vi "FlowPID.vi"() -> ()   [LabVIEW 2017]
uses:
  BERTTA.dll
panel:
  out "output2":dbl
  out "amount_out":dbl
  in  "flow_in":dbl
  out "errsum":i32
  out "Waveform Chart":dynamicdata(graph)
  out "error":i32
  out "output":i32
  out "timechange":i32
  out "lastTime":i32
  in  "kd":dbl
  in  "ki":dbl=1e-05
  in  "kp":dbl=0.001
  in  "Setpoint":dbl=2000.0
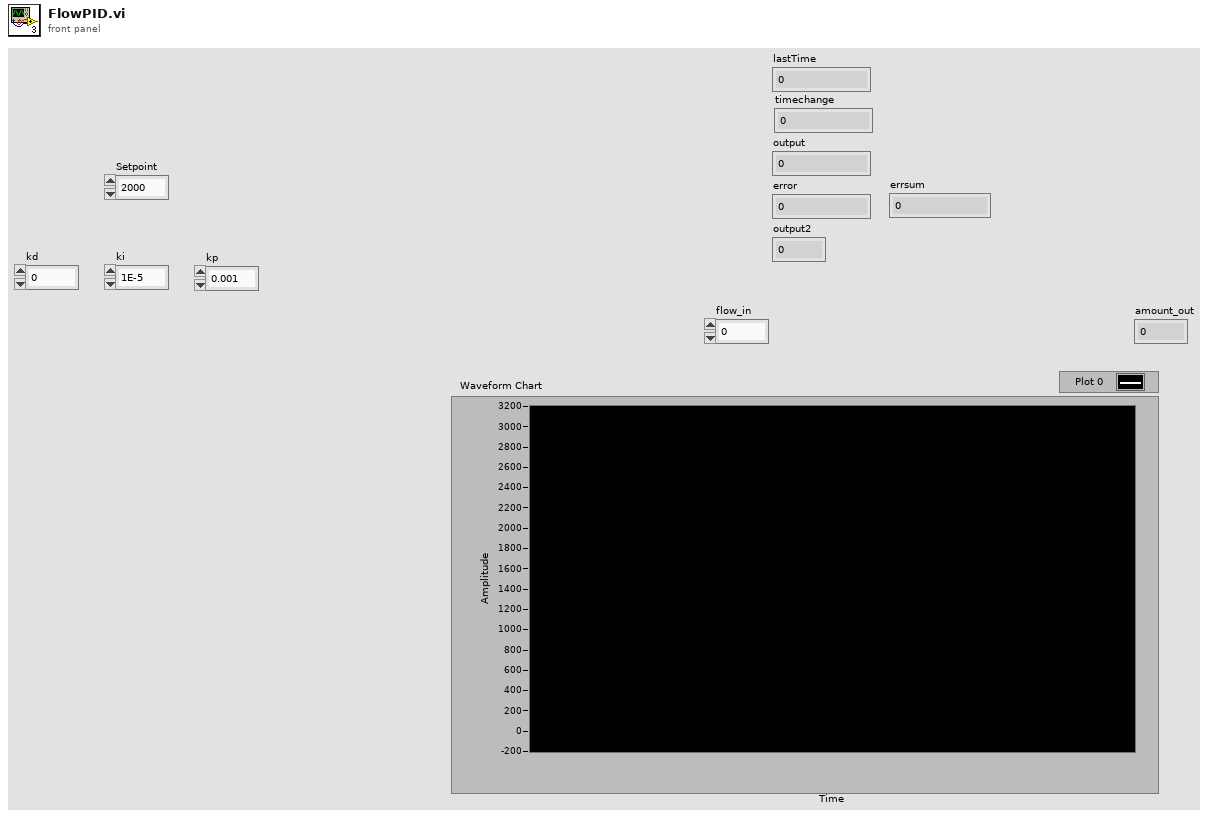
[diagram p1: front panel]
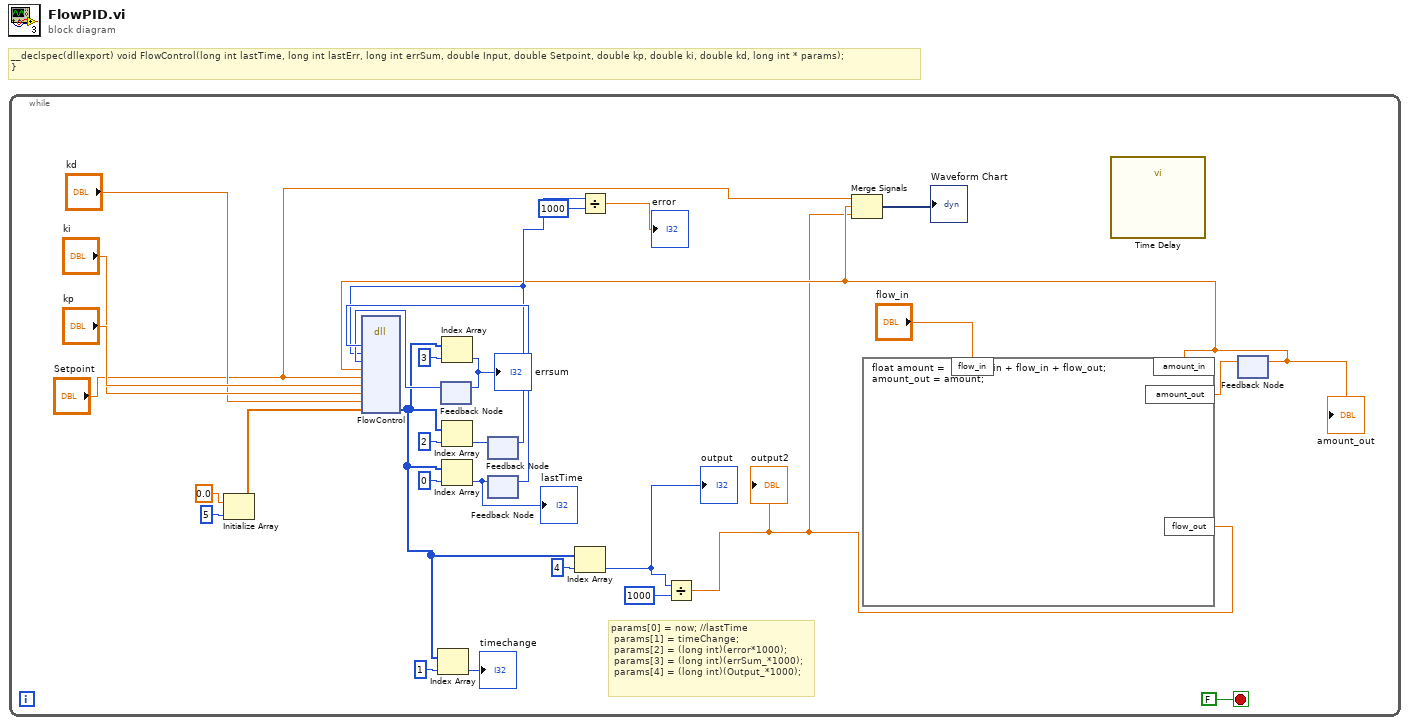
[diagram p0: block diagram]
diagram:
  # "__declspec(dllexport) void FlowControl(long int lastTime, long int lastErr, long int errSum, double Input, double Setpoint, double kp, double ki, double kd, long int * params);\n}"
  n1 = while {
    stop <- FALSE stop-if-true
    # "params[0] = now; //lastTime\n\tparams[1] = timeChange;\n\tparams[2] = (long int)(error*1000);\n\tparams[3] = (long int)(errSum_*1000);\n\tparams[4] = (long int)(Output_*1000);"
    n2 = Initialize Array(0.0 ("element"), 5 ("dimension size")) -> (w27:dbl[])
    n3 = feedback #1() -> (w14:i32)  [unwired: 1 in]
    n4 = feedback #2() -> (w11:i32)  [unwired: 1 in]
    n5 = feedback #3() -> (w20:i32)  [unwired: 1 in]
    n6 = Divide(x=w11, y=1000) -> (x/y=→"error":dbl)
    n7 = call "Time Delay"() -> ()  [unwired: 11 in, 1 out]
    n8 = feedback #4() -> (w3:dbl)  [unwired: 1 in]
    "amount_out" <- w3
    n9 = dll-call lib="C:/Users/p3cn/OneDrive - Kemira Oyj/Documents/GitHub/Bertta/BERTTA/x64/Release/BERTTA.dll" fn="FlowControl"("lastTime"=w20, "lastErr"=w11, "errSum"=w14, "Input"=w3, "Setpoint"="Setpoint", "kp"="kp", "ki"="ki", "kd"="kd", "PIDparams"=w27) -> ("PIDparams"=w12:i32[])  [unwired: 12 in, 2 out]
    n10 = Index Array(array=w12, index=1) -> (element=→"timechange":i32)
    n11 = Index Array(array=w12, index=3) -> (element=w15:i32)
    "errsum" <- w15
    n12 = feedback-in #1(w15) -> ()
    n13 = Index Array(array=w12, index=2) -> (element=w17:i32)
    n14 = Index Array(array=w12, index=0) -> (element=w21:i32)
    "lastTime" <- w21
    n15 = feedback-in #2(w17) -> ()
    n16 = feedback-in #3(w21) -> ()
    n17 = Index Array(array=w12, index=4) -> (element=w1:i32)
    "output" <- w1
    n18 = Divide(x=w1, y=1000) -> (x/y=w2:dbl)
    "output2" <- w2
    n19 = Merge Signals("Setpoint", w3, w2) -> (→"Waveform Chart":dynamicdata)
    n20 = formula code="float amount =  amount_in + flow_in + flow_out;\namount_out = amount;"("flow_in"="flow_in", "amount_in"=w3, "flow_out"=w2) -> ("amount_out"=w6:dbl)
    n21 = feedback-in #4(w6) -> ()
  }
